vi "AlliGator Unzip Python Plugins.vi"(8 "Error In":errorcluster, 11 "Application Directory":path) -> (0 "Error Out":errorcluster, 3 "Python Plugins Folder":path)   [LabVIEW 2021, in "AlliGator Python Plugins.lvlib"]
doc: "Unzips python plugin archive provided with AlliGator installation."
uses:
  AlliGator Python Plugins.lvlib
  AlliGator Settings List.ctl
  Variant/Variant to Data/Variant to String.vi
  AlliGator Globals.vi
  <userlib>/_OpenG.lib/lvzip/lvzip.llb/subVI/ZLIB Open Unzip Archive (Path)__ogtk.vi
  <userlib>/_OpenG.lib/lvzip/lvzip.llb/subVI/ZLIB Extract File (Path)__ogtk.vi
  AlliGator Settings.lvlib
  Variant/Variant to Data/Variant to Data.lvlib
  AlliGator Globals, Variables & Constants.lvlib
panel:
  out "Unmodified Files":path[](array[path])
  out "New Files":path[](array[path])
  # "see the AlliGator License on the block diagram (Ctrl+E or Window:Show Block Diagram)"
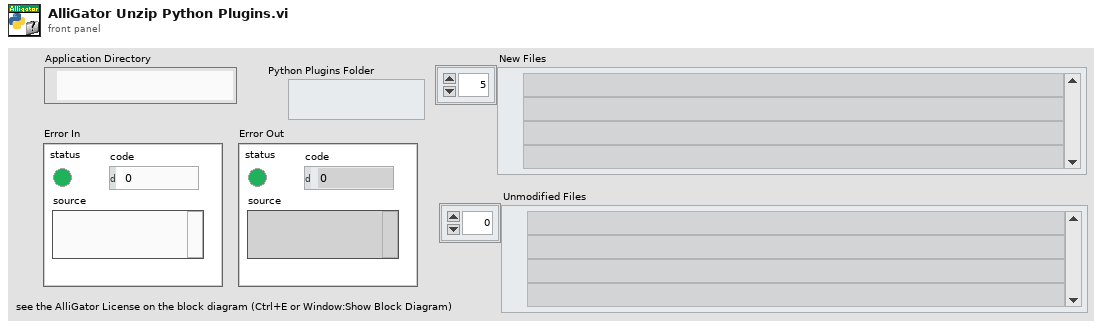
[diagram p1: front panel]
types:
  T1 = typedef "AlliGator Settings.lvlib/AlliGator Settings List.ctl" = enum16{"GUI:Visible Settings Tab", "GUI:Last Run Version", "Source Image:Use Image Histogram for Contrast", "Source Image:Low Count Pixels Rejection Options", "Source Image:High Count Pixels Rejection Options", "Source Image:Use Image Brightness", "Source Image:Blend Overlay with Image Background", "Source Image:Use Fixed ROI Diameter", "Source Image:ROI Diameter", "Source Image:ROI Center Color", "Source Image:Peak Threshold", "Source Image:Intensity Threshold", "Source Image:Image Binning Options", "Source Image:Image Smoothing Options", "Source Image:Image Histogram Active", "Source Image:Invert Binary Mask", "Source Image:Hot Pixel Removal", "Source Image:Overlay Analyzed ROI Center", "Source Image:Auto-Adjust Contrast", "Source Image:Histogram Lower Percentile", "Source Image:Histogram Upper Percentile", "Source Image:Save Source Image", "Source Image:Scale Bar Options", "Source Image:Image Resolution (Pixel Size)", "Source Image:Flatfield Correction", "Data Information:Gate Width", "Data Information:Nanotime Gate Separation", "Data Information:Macrotime Gate Separation", "Data Information:Gate Step", "Data Information:# Gates", "Data Information:Gate Image Exposure", "Data Information:Gate Image Integration", "Data Information:Gates to Skip", "Data Information:Gates to Keep", "Data Information:Define Gates to", "Data Information:Channel Name", "Data Information:Available Channel Names", "Data Information:Channel Arithmetic", "Data Information:Background File Subtraction", "Data Information:Background File", "Data Information:Background Scaling Factor", "Data Information:Background Pile-up Correction", "Data Information:Background Pixel Well Capacity", "Data Information:Laser Period", "Data Information:SYNC Period", "Data Information:Pile-up Correction", "Data Information:Pixel Well Capacity", "Data Information:Dataset Scaling Factor", "Fluorescence Decay_Decay Pre-Processing:Reverse Gates", "Fluorescence Decay_Decay Pre-Processing:Verbose Decay Pre-Processing", "Fluorescence Decay_Decay Pre-Processing:Use Decay Pre-Processing", "Fluorescence Decay_Decay Pre-Processing:Background Subtraction", "Fluorescence Decay_Decay Pre-Processing:Background Definition Range", "Fluorescence Decay_Decay Pre-Processing:Baseline Subtraction Method", "Fluorescence Decay_Decay Pre-Processing:Operations Order", "Fluorescence Decay_Decay Pre-Processing:Smoothing Parameter", "Fluorescence Decay_Decay Pre-Processing:Shift Decay", "Fluorescence Decay_Decay Pre-Processing:Decay Shift Parameters", "Fluorescence Decay_Decay Pre-Processing:Fold Decay", "Fluorescence Decay_Decay Pre-Processing:# Folds", "Fluorescence Decay_Decay Pre-Processing:1-Normalize Decay", "Fluorescence Decay_Decay Pre-Processing:[0-1]-Normalize Decay", "Fluorescence Decay_Decay Pre-Processing:Smoothen Decay", "Fluorescence Decay_Decay Pre-Processing:Extrapolate Decay", "Fluorescence Decay_Decay Pre-Processing:Use Periodicity", "Fluorescence Decay_Decay Pre-Processing:Use Cursors", "Fluorescence Decay_Decay Pre-Processing:Tail Fraction", "Fluorescence Decay_Decay Pre-Processing:Head Fraction", "Fluorescence Decay_Decay Pre-Processing:Additional Points", "Fluorescence Decay_Decay Pre-Processing:Straighten Decay", "Fluorescence Decay_Decay Pre-Processing:Constant Background", "Fluorescence Decay_Decay Pre-Processing:Pixel-Normalize Decay", "Fluorescence Decay_Advanced Analysis:Extract IRF instead of Decay", "Fluorescence Decay_Advanced Analysis:IRF Extraction Options", "Fluorescence Decay_Advanced Analysis:IRF Optimization Options", "Fluorescence Decay_Advanced Analysis:Square Pulse Options", "Fluorescence Decay_Advanced Analysis:IRF Order", "Fluorescence Decay_Advanced Analysis:IRF Time Constants", "Fluorescence Decay_Advanced Analysis:Wavelet Analysis Options", "Fluorescence Decay_Advanced Analysis:Average Lifetime Options", "Fluorescence Decay_Fit Options:Fit Options", "Fluorescence Decay_Fit Options:Use Legacy Fitting Approach", "Fluorescence Decay_Fit Options:Use Data Information Laser Period", "Fluorescence Decay_Fit Parameters:Displayed Fit Parameters", "Fluorescence Decay_Fit Parameters:Fit Parameter Constraints", "Fluorescence Decay_Fit Parameters:Export Tabulated Results", "Fluorescence Decay_Fit Parameters:MLE Baseline Offset Type", "Fluorescence Decay_Fit Parameters:MLE Baseline Offset", "Fluorescence Decay_Fit Parameters:Guess Parameter Names", "Fluorescence Decay_Fit Parameters:Guess Parameter Values", "Fluorescence Decay_Fit Parameters:Guess Parameters Options", "Fluorescence Decay_Styles:Show Last Decay Only", "Fluorescence Decay_Styles:Decay Graph Color Array", "Fluorescence Decay:Decay Graph Active", "Fluorescence Decay Statistics:Min Peak Value", "Fluorescence Decay Statistics:Reject Low Decay Peak Pixels", "Fluorescence Decay Statistics:Reject High Decay Peak Pixels", "Fluorescence Decay Statistics:Max Peak Value", "Time Traces:Use File Timestamp", "Time Traces:Time Step", "Time Traces:Use Intensity Correction File", "Time Traces:Intensity Correction File", "Phasor Plot:Phasor Plot Smoothing Options", "Phasor Plot:Phasor Plot Size", "Phasor Plot:Phasor Plot Graphics Options", "Phasor Plot:Cumulative Phasor Plot", "Phasor Plot:Use Phasor Brightness", "Phasor Plot:Blend Overlay with Phasor Background", "Phasor Plot:Save Phasor Plot", "Phasor Plot:Show References", "Phasor Plot:Phasor Ratio Decay Range", "Phasor Plot:Exponential Fading", "Phasor Plot:Phasor Ratio Reference Colors", "Phasor Plot:Reference Radius", "Phasor Plot:Show Color Map Vertices", "Phasor Plot:Phasor Plot Active", "Phasor Plot:Phasor Ratio Color Map Type", "Phasor Plot:Phasor Ratio Color Map", "Phasor Plot:Phasor Ratio Display Range", "Phasor Plot:Selected Image ROI(s)", "Phasor Plot:All Image ROIs", "Phasor Plot:Selected Phasor Plot ROI(s)", "Phasor Plot:All Phasor Plot ROIs", "Phasor Plot:Phasor Ratio Color-Coded Quantity", "Phasor Plot:Store Phasor Harmonics", "Phasor Plot:Draw Reference Segment", "Phasor Plot:User-Defined Quantity", "Phasor Graph:Phasor Frequency", "Phasor Graph:Phasor Ratio Type", "Phasor Graph:Pixel-level Phasor Computation", "Phasor Graph:Save Phasor Graph", "Phasor Graph:Phasor Graph Active", "Phasor Graph:Phasor SDV Options", "Phasor Calibration:Use Backup Calibration if needed", "Phasor Graph:Define Shortest Lifetime as", "Phasor Calibration:Backup Calibration Type", "Phasor Calibration:Calibration Type", "Phasor Calibration:Calibration Lifetime", "Phasor Calibration:Calibration Map Algorithm", "Single-Exponential Phasor Locus (SEPL):Gate Parameters", "Single-Exponential Phasor Locus (SEPL):User-defined Gate", "Single-Exponential Phasor Locus (SEPL):User-defined IRF", "Single-Exponential Phasor Locus (SEPL):Phasor Parameters", "Single-Exponential Phasor Locus (SEPL):Decay & IRF Parameters", "Single-Exponential Phasor Locus (SEPL):Display Parameters", "Lifetime Analysis:Decay Analysis Parameters", "Lifetime Analysis:Lifetime Map Active", "Plugins:Python Settings", "Miscellaneous:Verbose Mode", "Miscellaneous:Beep after Script", "Miscellaneous:Saved Image File Format", "Miscellaneous:Exported Gate Image Settings", "Miscellaneous:Include Loading in Timing", "Miscellaneous:Verbose Settings Mode", "Miscellaneous:Histogram Options", "Miscellaneous:Beep on Error", "Miscellaneous:# Logical Processors Used", "Miscellaneous:ROI Description Max Characters", "Miscellaneous:Verbose Error Mode", "Miscellaneous:Transparent Mask Color"}
  T2 = typedef "ZLIB Unzip Handle__ogtk.ctl" = refnum<k1>
  T3 = typedef "ZLIB File Info__ogtk.ctl" = cluster{"version":u32, "version needed":u32, "encrypted":bool, "flag":u32, "compression":i32, "dos date":u32, "crc":u32, "compressed size":i64, "uncompressed size":i64, "file comment":string, "disk num start":u32, "internal fa":u32, "external fa":u32, "file timestamp":u32, "extra info records":cluster{"id":u16, "data":u8[]}[]}
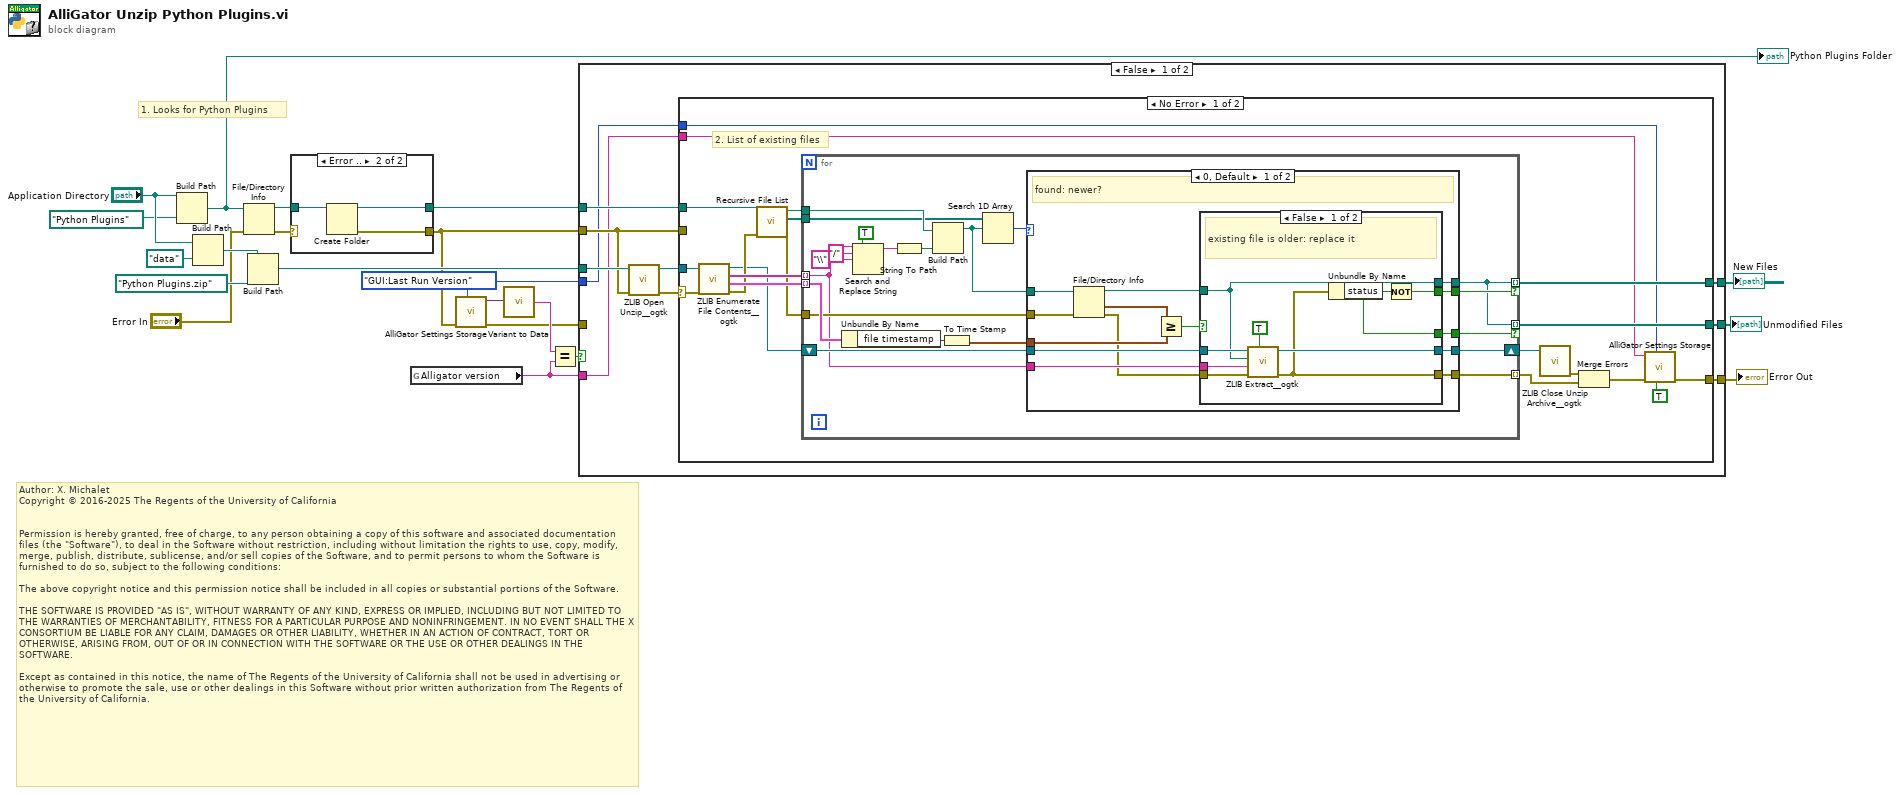
[diagram p0: block diagram]
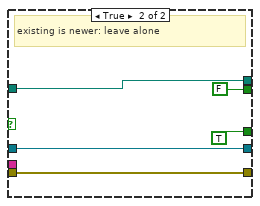
[diagram p2: hidden frame]
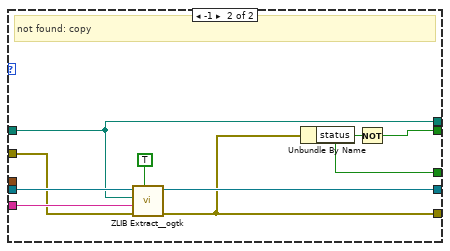
[diagram p3: hidden frame]
diagram:
  w2 = AlliGator_Settings_List."GUI:Last Run Version" ("AlliGator Settings List")
  # "Author: X. Michalet\nCopyright © 2016-2025 The Regents of the University of California\n \n\nPermission is hereby granted, free of charge, to any person obtaining a copy of this software and associated documentation files (the \"Software\"), to deal in the Software without restriction, including without limitation the rights to use, copy, modify, merge, publish, distribute, sublicense, and/or sell copies of the Software, and to permit persons to whom the Software is furnished to do so, subject to the following conditions:\n\nThe above copyright notice and this permission notice shall be included in all copies or substantial portions of the Software.\n\nTHE SOFTWARE IS PROVIDED \"AS IS\", WITHOUT WARRANTY OF ANY KIND, EXPRESS OR IMPLIED, INCLUDING BUT NOT LIMITED TO THE WARRANTIES OF MERCHANTABILITY, FITNESS FOR A PARTICULAR PURPOSE AND NONINFRINGEMENT. IN NO EVENT SHALL THE X CONSORTIUM BE LIABLE FOR ANY CLAIM, DAMAGES OR OTHER LIABILITY, WHETHER IN AN ACTION OF CONTRACT, TORT OR OTHERWISE, ARISING FROM, OUT OF OR IN CONNECTION WITH THE SOFTWARE OR THE USE OR OTHER DEALINGS IN THE SOFTWARE.\n\nExcept as contained in this notice, the name of The Regents of the University of California shall not be used in advertising or otherwise to promote the sale, use or other dealings in this Software without prior written authorization from The Regents of the University of California."
  # "1. Looks for Python Plugins"
  n1 = Build Path(base path="Application Directory", name or relative path=path "Python Plugins") -> (appended path=w8:path)
  "Python Plugins Folder" <- w8
  n2 = Build Path(base path="Application Directory", name or relative path=path "data") -> (appended path=w20:path)
  n3 = File/Directory Info(path=w8, error in="Error In") -> (path out=w16:path, error out=w17:errorcluster)  [unwired: 5 out]
  n4 = Build Path(base path=w20, name or relative path=path "Python Plugins.zip") -> (appended path=w13:path)
  n5 = case shown="Error .." w17 {
    selector: w17 -> [w22 _]
    tunnel: w16 -> [w23 w26]
    tunnel: [w23 w24] -> w12
    tunnel: [w22 w25] -> w7
    frame No Error {
    }
    frame Error {
      n6 = Create Folder(path (use dialog)=w26) -> (created path=w24:path, error out=w25:errorcluster)  [unwired: 2 in, 1 out]
    }
  }
  n7 = global read "AlliGator Globals.vi" "Alligator version"() -> (w1:string)
  n8 = call "AlliGator Settings Storage.vi"("AlliGator Settings List"=w2, "Error In"=w7) -> ("Error Out"=w3:errorcluster, "Variant Data out"=w6:variant)  [unwired: 8 in]
  n9 = call-poly "Variant to Data.vi"("Variant"=w6) -> ("String"=w5:string)  [unwired: 8 in]
  n10 = Equal?(x=w5, y=w1) -> (x = y?=w4:bool)
  n11 = case shown="False" w4 {
    tunnel: w13 -> [w34 _]
    tunnel: w12 -> [w33 _]
    tunnel: [w32 _] -> w11
    tunnel: [w31 _] -> w10
    tunnel: [w30 w115] -> w9
    tunnel: w7 -> [w29 _]
    tunnel: w3 -> [_ w115]
    tunnel: w2 -> [w28 _]
    tunnel: w1 -> [w27 _]
    frame False {
      n12 = call-poly <userlib>:"ZLIB Open Unzip__ogtk.vi"("error in (no error)"=w29, "archive name"=w34) -> ("error out"=w36:errorcluster, "unzip Refnum"=w35:T2)  [unwired: 4 in]
      n13 = case shown="No Error" w36 {
        selector: w36 -> [w54 _]
        tunnel: w35 -> [w53 _]
        tunnel: w33 -> [w51 _]
        tunnel: [w46 _] -> w32
        tunnel: [w44 _] -> w31
        tunnel: [w40 w114] -> w30
        tunnel: w29 -> [_ w114]
        tunnel: w28 -> [w39 _]
        tunnel: w27 -> [w38 _]
        frame No Error {
          # "2. List of existing files"
          n14 = call <userlib>:"ZLIB Enumerate File Contents__ogtk.vi"("error in (no error)"=w54, "unzip Refnum"=w53) -> ("error out"=w52:errorcluster, "file infos"=w56:T3[], "file names"=w55:string[], "unzip Refnum out"=w47:T2)  [unwired: 5 in, 1 out]
          n15 = call <vilib>:"Recursive File List.vi"("error in (no error)"=w52, "Folder Path"=w51) -> ("error out"=w48:errorcluster, "All Files in Dir"=w49:path[], "dup Folder Path"=w50:path)  [unwired: 5 in, 2 out]
          n16 = for {
            tunnel: w56 -> [w76] mode=indexing
            tunnel: w55 -> [w62] mode=indexing
            tunnel: w50 -> [w69]
            tunnel: w49 -> [w68]
            tunnel: w48 -> [w65]
            shift-right: [w61] -> w45
            shift-left: w47 -> [w63]
            tunnel: [w60] -> w42 mode=indexing
            tunnel: [w58] -> w46 mode=indexing if=w59
            tunnel: [w58] -> w44 mode=indexing if=w57
            n17 = Unbundle By Name(w76) -> ("file timestamp"=w75:u32)
            n18 = Search and Replace String(replace all?=TRUE ("replace all? (F)"), input string=w62, search string="/", replace string="\\" ("replace string (\"\")")) -> (result string=w74:string)  [unwired: 4 in, 3 out]
            n19 = String To Path(string=w74) -> (path=w70:path)
            n20 = Build Path(base path=w69, name or relative path=w70) -> (appended path=w66:path)
            n21 = To Time Stamp(1:w75) -> (0:w64:timestamp)
            n22 = Search 1D Array(1D array=w68, element=w66) -> (index of element=w67:i32)  [unwired: 1 in]
            n23 = case shown="0, Default" w67 {
              tunnel: w66 -> [w90 w106]
              tunnel: w65 -> [w89 w108]
              tunnel: [w85 w106] -> w58
              tunnel: [w84 w113] -> w59
              tunnel: [w83 w105] -> w57
              tunnel: w64 -> [w82 _]
              tunnel: w63 -> [w81 w112]
              tunnel: w62 -> [w80 w109]
              tunnel: [w78 w111] -> w61
              tunnel: [w77 w107] -> w60
              frame 0, Default {
                # "found: newer?"
                n24 = File/Directory Info(path=w90, error in=w89) -> (path out=w86:path, last mod=w88:timestamp, error out=w79:errorcluster)  [unwired: 4 out]
                n25 = Greater Or Equal?(x=w88, y=w82) -> (x >= y?=w87:bool)
                n26 = case shown="False" w87 {
                  tunnel: w86 -> [w94 w103]
                  tunnel: [w94 w103] -> w85
                  tunnel: [w92 FALSE] -> w84
                  tunnel: [w91 TRUE] -> w83
                  tunnel: w81 -> [w99 w100]
                  tunnel: w80 -> [w98 _]
                  tunnel: w79 -> [w97 w101]
                  tunnel: [w96 w100] -> w78
                  tunnel: [w93 w101] -> w77
                  frame False {
                    # "existing file is older: replace it"
                    n27 = call-poly <userlib>:"ZLIB Extract__ogtk.vi"("overwrite (F)"=TRUE, "error in (no error)"=w97, "internal name (same as target)"=w98, "target path"=w94, "unzip Refnum"=w99) -> ("error out"=w93:errorcluster, "unzip Refnum out"=w96:T2)  [unwired: 2 in, 1 out]
                    n28 = Unbundle By Name(w93) -> ("status"=w91:bool)
                    n29 = Not(x=w91) -> (.not. x?=w92:bool)
                  }
                  frame True {
                    # "existing is newer: leave alone"
                  }
                }
              }
              frame -1 {
                # "not found: copy"
                n30 = call-poly <userlib>:"ZLIB Extract__ogtk.vi"("overwrite (F)"=TRUE, "error in (no error)"=w108, "internal name (same as target)"=w109, "target path"=w106, "unzip Refnum"=w112) -> ("error out"=w107:errorcluster, "unzip Refnum out"=w111:T2)  [unwired: 2 in, 1 out]
                n31 = Unbundle By Name(w107) -> ("status"=w105:bool)
                n32 = Not(x=w105) -> (.not. x?=w113:bool)
              }
            }
          }
          n33 = call <userlib>:"ZLIB Close Unzip Archive__ogtk.vi"("unzip Refnum"=w45) -> ("error out"=w43:errorcluster)  [unwired: 5 in, 1 out]
          n34 = Merge Errors(w43, w42) -> (w41:errorcluster)
          n35 = call "AlliGator Settings Storage.vi"("Get(F)/Set"=TRUE, "AlliGator Settings List"=w39, "Error In"=w41, "Variant Data in"=w38) -> ("Error Out"=w40:errorcluster)  [unwired: 6 in, 1 out]
        }
        frame Error {
        }
      }
    }
    frame True {
      # "Not the first run: do not overwrite Plugins folder"
    }
  }
  "Error Out" <- w9
  "New Files" <- w11
  "Unmodified Files" <- w10
